vi "Verify g-cli.vi"(8 "error in":errorcluster) -> (0 "error out":errorcluster)   [LabVIEW 2026, in "Caraya Extension Tests.lvclass"]
uses:
  Caraya Extension Tests.lvclass
  Caraya Extension Tests.lvclass/Caraya Extension Tests.ctl
  <vilib>/addons/_JKI Toolkits/Caraya/classes/Test/Test.lvclass
  Source/Extensions/Caraya.Extension/Caraya.Extension.lvlib
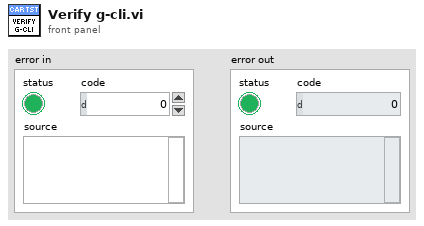
[diagram p1: front panel]
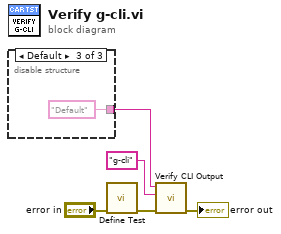
[diagram p0: block diagram]
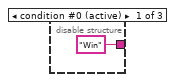
[diagram p2: hidden frame]
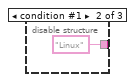
[diagram p3: hidden frame]
diagram:
  n1 = disable-structure shown="Default" {
    disable-tunnel: ["Win" ("Label") "Linux" ("Label") "Default" ("Label")] -> w1
    frame condition #0 (active) {
    }
    frame condition #1 {
    }
    frame condition #2 {
    }
  }
  n2 = call <vilib>:"Define Test.vi"("error in (no error)"="error in") -> ("error out"=w3:errorcluster)  [unwired: 9 in, 1 out]
  n3 = call "Verify CLI Output.vi"("error in"=w3, "command line"="g-cli", "Label"=w1) -> ("error out"=→"error out":errorcluster)  [unwired: 7 in, 1 out]
